vi "随机数发生器（韦伯分布）.vi"(3 "Gamma":dbl, 4 "Alpha(>0)":dbl, 5 "Beta(>0)":dbl, 6 "Num":i32) -> (1 "x":dbl[](array[numeric]))   [LabVIEW 2012]
doc: "功能：\n\n产生系列符合韦伯分布的随机变量。\n\n\n\n\n\ncsxcs_366创建"
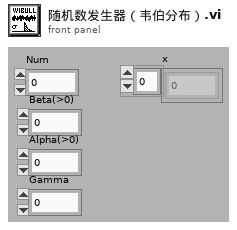
[diagram p1: front panel]
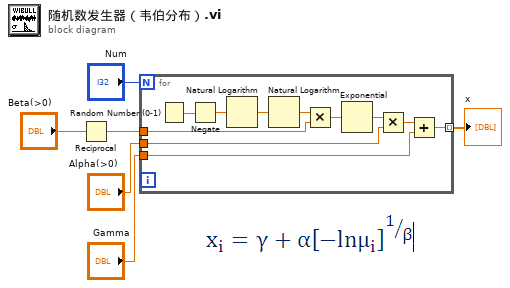
[diagram p0: block diagram]
diagram:
  n1 = Reciprocal(x="Beta(>0)") -> (1/x=w4:dbl)
  n2 = for {
    N: "Num" -> [_]
    tunnel: w4 -> [w13]
    tunnel: "Alpha(>0)" -> [w10]
    tunnel: "Gamma" -> [w8]
    tunnel: [w7] -> w1 mode=indexing
    n3 = Random Number (0-1)() -> (number: 0 to 1=w17:dbl)
    n4 = Negate(x=w17) -> (-x=w16:dbl)
    n5 = Natural Logarithm(1:w16) -> (0:w15:dbl)
    n6 = Natural Logarithm(1:w15) -> (0:w14:dbl)
    n7 = Multiply(x=w14, y=w13) -> (x*y=w12:dbl)
    n8 = Exponential(1:w12) -> (0:w11:dbl)
    n9 = Multiply(x=w11, y=w10) -> (x*y=w9:dbl)
    n10 = Add(x=w9, y=w8) -> (x+y=w7:dbl)
  }
  "x" <- w1
